vi "Count displayable text lines.vi"(4 "Original String Reference In":refnum<vi>) -> (1 "Number of lines":u32)   [LabVIEW 2014]
doc: "This VI will count the number of lines displayable in a text control."
panel:
  in  "local string":string
  # "This VI will count the number of lines displayable\nin a text control."
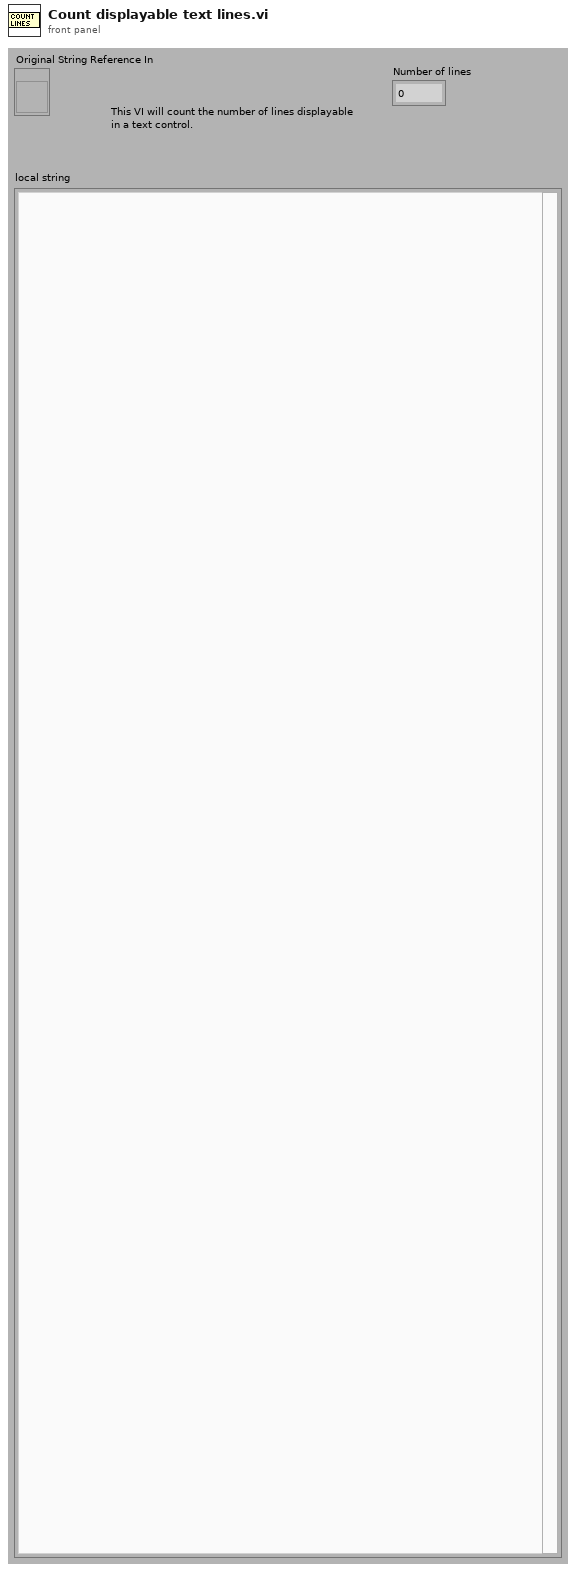
[diagram p1: front panel]
types:
  T1 = typedef "LVFontTypeDef.ctl" = cluster{"Font Name":string, "Size":u16, "Bold":bool, "Italic":bool, "Underline":bool, "Strikeout":bool, "Color":u32}
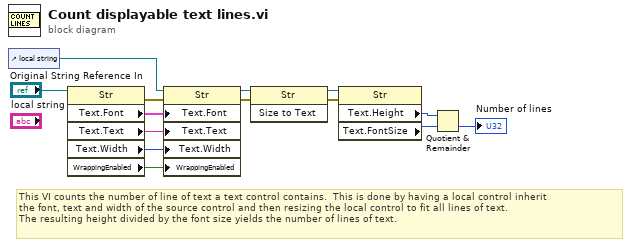
[diagram p0: block diagram]
diagram:
  # "This VI counts the number of line of text a text control contains.  This is done by having a local control inherit\nthe font, text and width of the source control and then resizing the local control to fit all lines of text.\nThe resulting height divided by the font size yields the number of lines of text."
  n1 = control-ref of="local string"() -> (w10:refnum<vi>)
  n2 = property class="Str"(reference="Original String Reference In") -> (error out=w13:errorcluster, "Text.Font"=w12:T1, "Text.Text"=w11:string, "Text.Width"=w9:u32, "WrappingEnabled"=w1:bool)  [unwired: 1 in, 1 out]
  n3 = property class="Str"(reference=w10, error in=w13, "Text.Font"=w12, "Text.Text"=w11, "Text.Width"=w9, "WrappingEnabled"=w1) -> (reference out=w8:refnum<vi>, error out=w7:errorcluster)
  n4 = invoke class="Str" method="Size to Text"(reference=w8, error in=w7) -> (reference out=w6:refnum<vi>, error out=w5:errorcluster)  [unwired: 1 in, 1 out]
  n5 = property class="Str"(reference=w6, error in=w5) -> ("Text.Height"=w3:u32, "Text.FontSize"=w4:u32)  [unwired: 2 out]
  n6 = Quotient & Remainder(x=w3, y=w4) -> (floor(x/y)=→"Number of lines":u32)  [unwired: 1 out]
